vi "FGV_HovaCAL_Interface_Kommandos.vi"(5 "Aktion":T2, 7 "error in":errorcluster, 9 "connected in ?":bool, 10 "Kommando in":T1) -> (0 "error out":errorcluster, 1 "Kommandos gesammelt":T1[](array[typedef]), 2 "Kommandos out":T1[](array[typedef]), 3 "Kommando out":T1, 4 "gesammelt ?":bool, 6 "connected out ?":bool)   [LabVIEW 2020, in "Linearisierung v2.lvlib" / "Gasteiler.lvlib" / "HovaCAL_Interface.lvlib" / "Kommunikation.lvlib"]
uses:
  Kommunikation.lvlib
  Aktion_FGV_HovaCAL_Interface_Kommandos.ctl
  Aktion_FGV_HovaCAL_Interface_Kommunikation.ctl
  Aktion_FGV_HovaCAL_Interface_GetData.ctl
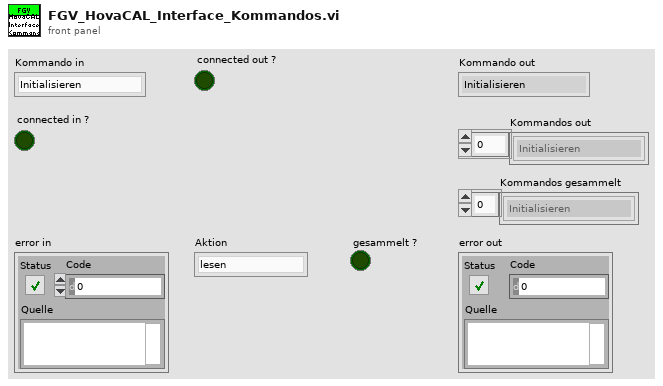
[diagram p1: front panel]
types:
  T1 = typedef "Linearisierung v2.lvlib/Gasteiler.lvlib/HovaCAL_Interface.lvlib/Kommunikation.lvlib/Aktion_FGV_HovaCAL_Interface_Kommunikation.ctl" = enum16{"Initialisieren", "Set Konzentrationen", "Set Gase", "Set Limits", "Get Dynamische Werte", "Beenden", "Com ändern", "Get Gase init", "Pause", "Get Gasteiler Infos", "Get MFC Infos", "Set Pumpen Parameter", "Set Pumpe Konzenration", "Set Pumpe run", "Set Temperaturen", "Set Fluss", "Get Gase", "Get Limits", "Get Dynamische Werte 1", "Get Dynamische Werte 2"}
  T2 = typedef "Linearisierung v2.lvlib/Gasteiler.lvlib/HovaCAL_Interface.lvlib/Kommunikation.lvlib/Aktion_FGV_HovaCAL_Interface_Kommandos.ctl" = enum16{"lesen", "verarbeiten", "hinzufügen", "on top", "init", "sammeln", "freigeben", "connected"}
  T3 = cluster{"first contact in":bool, "first actual values in ":bool}
  T4 = typedef "Linearisierung v2.lvlib/Gasteiler.lvlib/HovaCAL_Interface.lvlib/Kommunikation.lvlib/Aktion_FGV_HovaCAL_Interface_GetData.ctl" = enum16{"lesen", "SystemInfo", "MFC Info", "actual Values", "Limits", "first contact", "reset after read"}
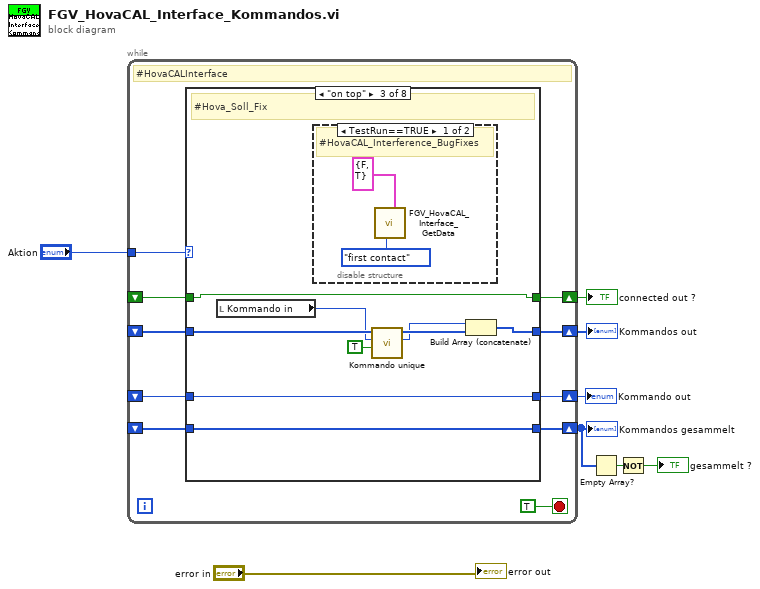
[diagram p0: block diagram]
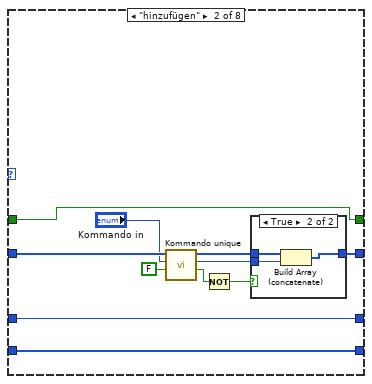
[diagram p3: hidden frame]
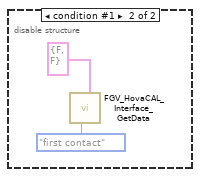
[diagram p5: hidden frame]
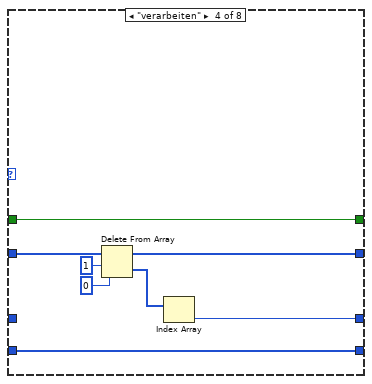
[diagram p6: hidden frame]
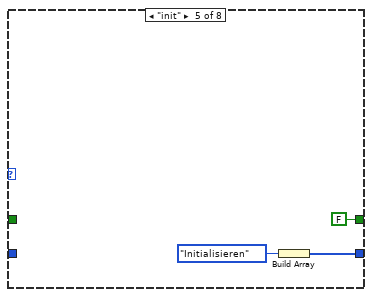
[diagram p7: hidden frame]
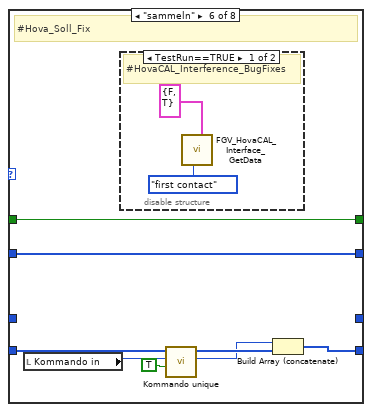
[diagram p8: hidden frame]
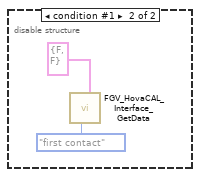
[diagram p9: hidden frame]
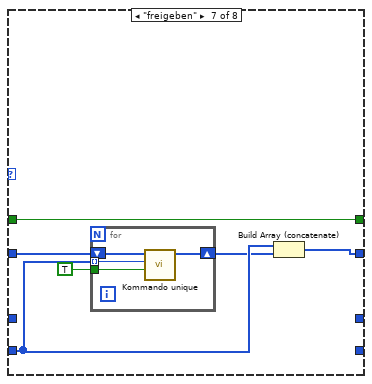
[diagram p10: hidden frame]
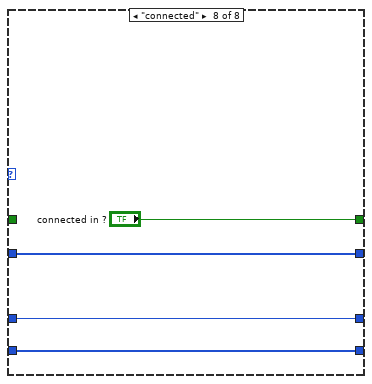
[diagram p11: hidden frame]
diagram:
  n1 = while {
    tunnel: "Aktion" -> [w18]
    shift-right: [w16] -> w7
    shift-left: _ -> [w15]
    shift-right: [w14] -> w6
    shift-left: _ -> [w13]
    shift-right: [w12] -> w4
    shift-left: _ -> [w11]
    shift-right: [w10] -> w1
    shift-left: _ -> [w9]
    stop <- TRUE stop-if-true
    # "#HovaCALInterface"
    n2 = case shown="\"on top\"" w18 {
      tunnel: [w22 w32 w45 w57 w60 w69 w79 w87] -> w16
      tunnel: w15 -> [w22 w31 w44 w58 _ w69 w77 w87]
      tunnel: [w21 w33 w46 w53 _ _ _ w84] -> w14
      tunnel: w13 -> [w21 w33 w46 _ _ _ _ w84]
      tunnel: [w20 w24 w39 w52 _ w68 _ w86] -> w12
      tunnel: w11 -> [w20 w24 w39 w52 _ w64 w78 w86]
      tunnel: [w19 w23 w38 w51 FALSE ("connected in ?") w62 w74 "connected in ?"] -> w10
      tunnel: w9 -> [w19 w23 w38 w51 _ w62 w74 _]
      frame "lesen", Default {
      }
      frame "hinzufügen" {
        n3 = call "Kommando unique.vi"("remove"=FALSE, "Kommando in (Eingang)"="Kommando in", "Array (Eingang)"=w31) -> ("found"=w27:bool, "Kommando out"=w28:T1, "Array (Ausgang)"=w30:T1[])  [unwired: 6 in]
        n4 = Not(x=w27) -> (.not. x?=w26:bool)
        n5 = case shown="True" w26 {
          tunnel: [w34 w37] -> w32
          tunnel: w30 -> [w34 w36]
          tunnel: w28 -> [_ w35]
          frame False {
          }
          frame True {
            n6 = Build Array (concatenate)(w36, w35) -> (w37:T1[])
          }
        }
      }
      frame "on top" {
        # "#Hova_Soll_Fix"
        n7 = local read "Kommando in"() -> (w41:T1)
        n8 = disable-structure shown="TestRun==TRUE" {
          frame condition #0 (active) {
            # "#HovaCAL_Interference_BugFixes"
            n9 = call "FGV_HovaCAL_Interface_GetData.vi"("first flags in"=T3 {"first contact in"=FALSE, "first actual values in "=TRUE}, "Aktion"=Aktion_FGV_HovaCAL_Interface_GetData."first contact") -> ()  [unwired: 5 in, 5 out]
          }
          frame condition #1 {
            n10 = call "FGV_HovaCAL_Interface_GetData.vi"("first flags in"=T3 {"first contact in"=FALSE, "first actual values in "=FALSE}, "Aktion"=Aktion_FGV_HovaCAL_Interface_GetData."first contact") -> ()  [unwired: 5 in, 5 out]
          }
        }
        n11 = call "Kommando unique.vi"("remove"=TRUE, "Kommando in (Eingang)"=w41, "Array (Eingang)"=w44) -> ("Kommando out"=w40:T1, "Array (Ausgang)"=w43:T1[])  [unwired: 6 in, 1 out]
        n12 = Build Array (concatenate)(w40, w43) -> (w45:T1[])
      }
      frame "verarbeiten" {
        n13 = Delete From Array(array=w58, length=1 ("Länge"), index=0 ("Index")) -> (deleted portion=w54:T1[], array with subset deleted=w57:T1[])
        n14 = Index Array(array=w54) -> (element=w53:T1)  [unwired: 1 in]
      }
      frame "init" {
        n15 = Build Array(Aktion_FGV_HovaCAL_Interface_Kommunikation."Initialisieren" ("Kommando")) -> (w60:T1[])
      }
      frame "sammeln" {
        # "#Hova_Soll_Fix"
        n16 = local read "Kommando in"() -> (w66:T1)
        n17 = disable-structure shown="TestRun==TRUE" {
          frame condition #0 (active) {
            # "#HovaCAL_Interference_BugFixes"
            n18 = call "FGV_HovaCAL_Interface_GetData.vi"("first flags in"=T3 {"first contact in"=FALSE, "first actual values in "=TRUE}, "Aktion"=Aktion_FGV_HovaCAL_Interface_GetData."first contact") -> ()  [unwired: 5 in, 5 out]
          }
          frame condition #1 {
            n19 = call "FGV_HovaCAL_Interface_GetData.vi"("first flags in"=T3 {"first contact in"=FALSE, "first actual values in "=FALSE}, "Aktion"=Aktion_FGV_HovaCAL_Interface_GetData."first contact") -> ()  [unwired: 5 in, 5 out]
          }
        }
        n20 = call "Kommando unique.vi"("remove"=TRUE, "Kommando in (Eingang)"=w66, "Array (Eingang)"=w64) -> ("Kommando out"=w63:T1, "Array (Ausgang)"=w65:T1[])  [unwired: 6 in, 1 out]
        n21 = Build Array (concatenate)(w63, w65) -> (w68:T1[])
      }
      frame "freigeben" {
        n22 = for {
          tunnel: w78 -> [w83] mode=indexing
          shift-right: [w82] -> w76
          shift-left: w77 -> [w81]
          tunnel: TRUE ("remove") -> [w80]
          n23 = call "Kommando unique.vi"("remove"=w80, "Kommando in (Eingang)"=w83, "Array (Eingang)"=w81) -> ("Array (Ausgang)"=w82:T1[])  [unwired: 6 in, 2 out]
        }
        n24 = Build Array (concatenate)(w78, w76) -> (w79:T1[])
      }
      frame "connected" {
      }
    }
  }
  "Kommandos out" <- w7
  "Kommando out" <- w6
  "Kommandos gesammelt" <- w4
  "connected out ?" <- w1
  n25 = Empty Array?(array=w4) -> (empty?=w3:bool)
  n26 = Not(x=w3) -> (.not. x?=→"gesammelt ?":bool)
  "error out" <- "error in"
